vi "Local IA Control.vi"(9 "E-Stop Vacuum":bool=TRUE, 10 "Irrigate?":bool=TRUE, 11 "8bit integer":i8) -> (1 "Accurus Engaged Vout":dbl, 2 "Accurus ChB Vout":dbl, 3 "Accurus ChA Vout":dbl)   [LabVIEW 2016]
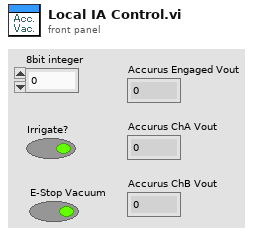
[diagram p1: front panel]
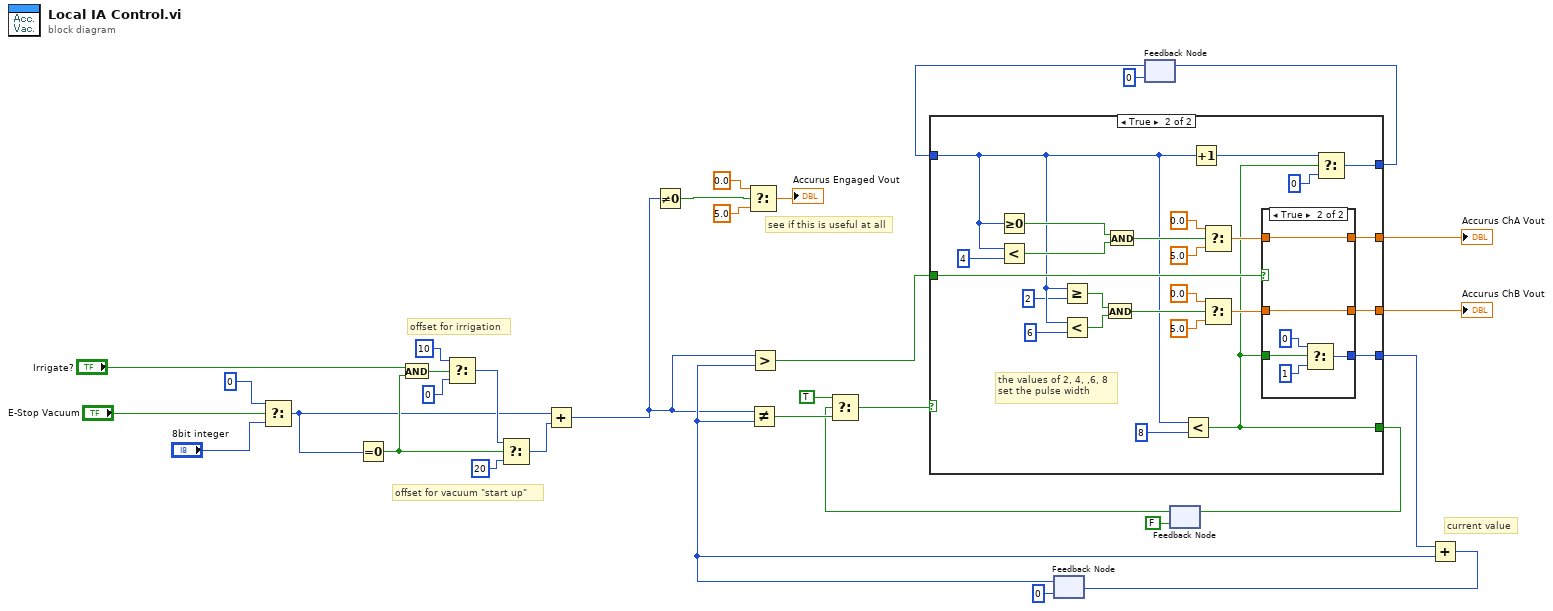
[diagram p0: block diagram]
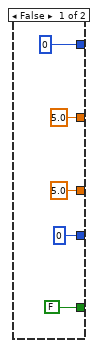
[diagram p2: hidden frame]
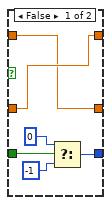
[diagram p3: hidden frame]
diagram:
  # "see if this is useful at all"
  # "offset for irrigation"
  # "offset for vacuum \"start up\""
  # "current value"
  n1 = Select(t=i8 0, s="E-Stop Vacuum", f="8bit integer") -> (s? t:f=w4:i8)
  n2 = Equal To 0?(x=w4) -> (x = 0?=w11:bool)
  n3 = And(x="Irrigate?", y=w11) -> (x .and. y?=w10:bool)
  n4 = Select(t=i8 10, s=w10, f=i8 0 ("t")) -> (s? t:f=w6:i8)
  n5 = Select(t=w6, s=w11, f=i8 20) -> (s? t:f=w31:i8)
  n6 = Add(x=w4, y=w31) -> (x+y=w5:i8)
  n7 = Not Equal To 0?(x=w5) -> (x != 0?=w7:bool)
  n8 = Select(t=0.0, s=w7, f=5.0) -> (s? t:f=→"Accurus Engaged Vout":dbl)
  n9 = feedback #1(i8 0) -> (w18:i8)
  n10 = Not Equal?(x=w5, y=w18) -> (x != y?=w24:bool)
  n11 = Greater?(x=w5, y=w18) -> (0:w14:bool)
  n12 = feedback #2(i8 0) -> (w20:i8)
  n13 = feedback #3(FALSE) -> (w21:bool)
  n14 = Select(t=TRUE, s=w21, f=w24) -> (s? t:f=w23:bool)
  n15 = case shown="True" w23 {
    tunnel: [5.0 ("f") w51] -> w28
    tunnel: [5.0 ("f") w50] -> w29
    tunnel: [i8 0 ("f") w48] -> w17
    tunnel: [FALSE w43] -> w13
    tunnel: w14 -> [_ w49]
    tunnel: [i8 0 w45] -> w15
    tunnel: w20 -> [_ w47]
    frame False {
    }
    frame True {
      # "the values of 2, 4, ,6, 8 \nset the pulse width"
      n16 = Greater Or Equal To 0?(x=w47) -> (x >= 0?=w58:bool)
      n17 = Less?(x=w47, y=i8 4) -> (x < y?=w57:bool)
      n18 = Greater Or Equal?(x=w47, y=i8 2) -> (x >= y?=w56:bool)
      n19 = Less?(x=w47, y=i8 6) -> (x < y?=w55:bool)
      n20 = And(x=w56, y=w55) -> (x .and. y?=w54:bool)
      n21 = And(x=w58, y=w57) -> (x .and. y?=w59:bool)
      n22 = Less?(x=w47, y=i8 8) -> (x < y?=w43:bool)
      n23 = Increment(x=w47) -> (x+1=w46:i8)
      n24 = Select(t=0.0, s=w59, f=5.0) -> (s? t:f=w53:dbl)
      n25 = Select(t=0.0, s=w54, f=5.0) -> (s? t:f=w52:dbl)
      n26 = case shown="True" w49 {
        tunnel: w53 -> [w68 w74]
        tunnel: w52 -> [w69 w75]
        tunnel: [w68 w75] -> w50
        tunnel: [w69 w74] -> w51
        tunnel: w43 -> [w64 w73]
        tunnel: [w65 w72] -> w48
        frame False {
          n27 = Select(t=i8 0, s=w64, f=i8 -1) -> (s? t:f=w65:i8)
        }
        frame True {
          n28 = Select(t=i8 0, s=w73, f=i8 1) -> (s? t:f=w72:i8)
        }
      }
      n29 = Select(t=w46, s=w43, f=i8 0) -> (s? t:f=w45:i8)
    }
  }
  "Accurus ChB Vout" <- w29
  "Accurus ChA Vout" <- w28
  n30 = feedback-in #2(w15) -> ()
  n31 = feedback-in #3(w13) -> ()
  n32 = Add(x=w17, y=w18) -> (x+y=w33:i8)
  n33 = feedback-in #1(w33) -> ()
